vi "Global.vi"() -> ()   [LabVIEW 2018]
panel:
  in  "Stop":bool
  in  "Knob":dbl(knob) scale=0.0..10.0
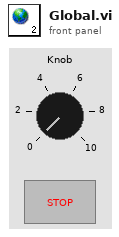
[diagram p1: front panel]
diagram:
